vi "LEDs_ON.vi"(8 "error in (no error)":errorcluster, 11 "channel":refnum<k24>) -> (0 "error out":errorcluster)   [LabVIEW 2021]
uses:
  F:/2PhotonVision/psychometric_function_v2/lib/Grpc.Core.dll
  lib/Grpc.Core.dll
  F:/2PhotonVision/psychometric_function_v2/lib/FossilProtosSharp.dll
  lib/FossilProtosSharp.dll
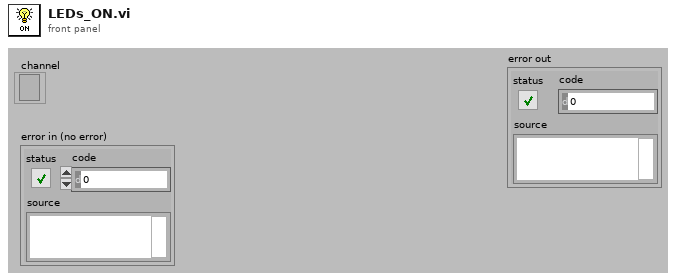
[diagram p1: front panel]
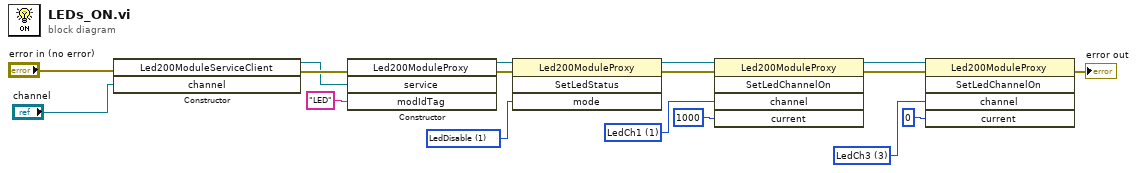
[diagram p0: block diagram]
diagram:
  w16 = 3 items=["LedChUnspecified", "LedCh1", "LedCh2", "LedCh3", "LedCh4"] ("channel")
  w12 = 1 items=["LedChUnspecified", "LedCh1", "LedCh2", "LedCh3", "LedCh4"] ("channel")
  w8 = 1 items=["LedUnspecified", "LedDisable", "LedEnable", "LedOnlyErrors", "LedStatus"] ("mode")
  n1 = constructor class="Led200ModuleServiceClient"(error in="error in (no error)", "channel"="channel") -> (reference out=w3:refnum<k24>, error out=w4:errorcluster)  [unwired: 2 in, 2 out]
  n2 = constructor class="Led200ModuleProxy"(error in=w4, "service"=w3, "modIdTag"="LED") -> (reference out=w7:refnum<k24>, error out=w9:errorcluster)  [unwired: 2 in, 3 out]
  n3 = invoke class="Led200ModuleProxy" method="SetLedStatus"(reference=w7, error in=w9, "mode"=w8) -> (reference out=w10:refnum<k24>, error out=w14:errorcluster)  [unwired: 1 in, 2 out]
  n4 = invoke class="Led200ModuleProxy" method="SetLedChannelOn"(reference=w10, error in=w14, "channel"=w12, "current"=1000) -> (reference out=w11:refnum<k24>, error out=w15:errorcluster)  [unwired: 1 in, 3 out]
  n5 = invoke class="Led200ModuleProxy" method="SetLedChannelOn"(reference=w11, error in=w15, "channel"=w16, "current"=0) -> (error out=→"error out":errorcluster)  [unwired: 1 in, 4 out]
